vi "Graphics-Transparency Mask to Boolean Matrix.vi"(9 "Columns":i32, 10 "Rows":i32, 11 "Mask In":u8[](array[numeric])) -> (3 "Mask Out":bool[][](array[boolean]))   [LabVIEW 2015]
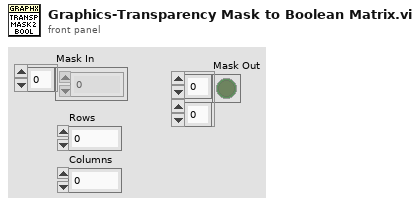
[diagram p1: front panel]
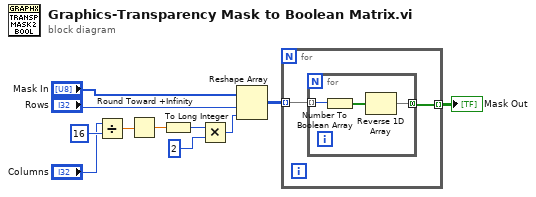
[diagram p0: block diagram]
diagram:
  n1 = Divide(x="Columns", y=16) -> (x/y=w9:dbl)
  n2 = Round Toward +Infinity(x=w9) -> (ceil(x): smallest int >= x=w8:dbl)
  n3 = To Long Integer(number=w8) -> (32bit integer=w6:i32)
  n4 = Multiply(x=w6, y=2) -> (x*y=w2:i32)
  n5 = Reshape Array("Mask In", "Rows", w2) -> (w5:u8[][])
  n6 = for {
    tunnel: w5 -> [w13] mode=indexing
    tunnel: [w12] -> w3 mode=indexing
    n7 = for {
      tunnel: w13 -> [w16] mode=indexing
      tunnel: [w14] -> w12 mode=concatenating
      n8 = Number To Boolean Array(number=w16) -> (Boolean array=w15:bool[])
      n9 = Reverse 1D Array(array=w15) -> (reversed array=w14:bool[])
    }
  }
  "Mask Out" <- w3
